vi "Set Timeout.vi"(8 "error in (no error)":errorcluster, 10 "Timeout Period in ms (-1, never)":i32=-1, 11 "State Machine Actor in":refnum<class "State Machine Actor.lvclass">) -> (0 "error out":errorcluster, 3 "State Machine Actor out":refnum<class "State Machine Actor.lvclass">)   [LabVIEW 2024, in "State Machine Actor.lvlib" / "State Machine Actor.lvclass"]
uses:
  State Machine Actor.lvclass
  State Machine Actor.lvclass/State Machine Actor.ctl
  <vilib>/ActorFramework/Actor/Actor.lvclass
  State Machine Actor Messages/Timeout Msg/Timeout Msg.lvclass
  C:/Users/uspoaotto/OneDrive - Oregon Tool/Desktop/working copies/stateMachineActor/src/_State Machine Actor/_State Machine Actor/_State Machine Actor.lvclass
  C:/Program Files (x86)/National Instruments/LabVIEW 2024/vi.lib/ActorFramework/Actor/Actor.lvclass
  C:/Users/uspoaotto/OneDrive - Oregon Tool/Desktop/working copies/stateMachineActor/src/State Machine Actor/State Machine Actor/State Machine Actor.lvclass
  C:/Program Files (x86)/National Instruments/LabVIEW 2024/vi.lib/ActorFramework/Message/Message.lvclass
  C:/Users/uspoaotto/OneDrive - Oregon Tool/Desktop/working copies/stateMachineActor/src/State Machine Actor/State Machine Actor Messages/Timeout Msg/Timeout Msg.lvclass
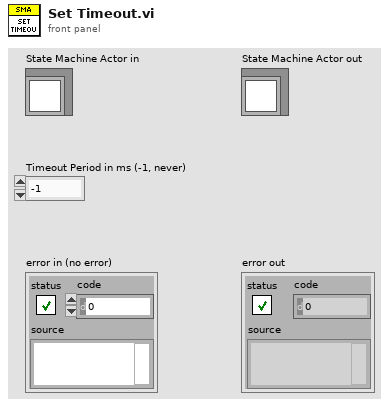
[diagram p1: front panel]
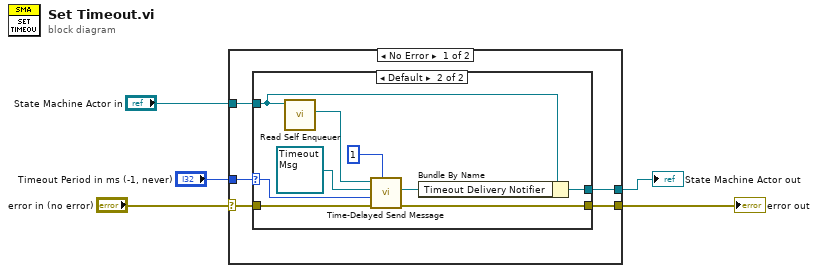
[diagram p0: block diagram]
diagram:
  n1 = case shown="No Error" "error in (no error)" {
    selector: "error in (no error)" -> [w9 w23]
    tunnel: [w8 w23] -> w4
    tunnel: [w7 w22] -> w2
    tunnel: "State Machine Actor in" -> [w10 w22]
    tunnel: "Timeout Period in ms (-1, never)" -> [w6 _]
    frame No Error {
      n2 = case shown="Default" w6 {
        selector: w6 -> [_ w20]
        tunnel: [w11 w18] -> w7
        tunnel: [w12 w17] -> w8
        tunnel: w10 -> [w11 w14]
        tunnel: w9 -> [w12 w15]
        frame -1 {
        }
        frame Default {
          n3 = call <vilib>:"Read Self Enqueuer.vi"("Actor"=w14) -> ("Self Enqueuer"=w16:refnum<class "Message Enqueuer.lvclass">)  [unwired: 10 in]
          n4 = call <vilib>:"Time-Delayed Send Message.vi"("# Copies (0 = infinite repeat)"=u32 1, "error in (no error)"=w15, "Milliseconds To Wait"=w20, "Message"=refnum<class "Timeout Msg.lvclass"> refnum ("State Machine Actor.lvlib:Timeout Msg.lvclass"), "Message Enqueuer"=w16) -> ("error out"=w17:errorcluster, "Delivery Notifier"=w19:refnum<notifier>)  [unwired: 5 in]
          n5 = Bundle By Name(cluster=w14, "Timeout Delivery Notifier"=w19) -> (w18:refnum<class "State Machine Actor.lvclass">)
        }
      }
    }
    frame Error {
    }
  }
  "error out" <- w4
  "State Machine Actor out" <- w2
